vi "周期设置_采配水.vi"() -> ()   [LabVIEW 2016, in "环境动力单元.lvlib"]
uses:
  <vilib>/Utility/miscctls.llb/LVPointTypeDef.ctl
  <vilib>/Utility/config.llb/NI_LVConfig.lvlib
  <vilib>/ptbypt/NI_PtbyPt.lvlib
panel:
  in  "运行周期":T1
  # "运行模式："
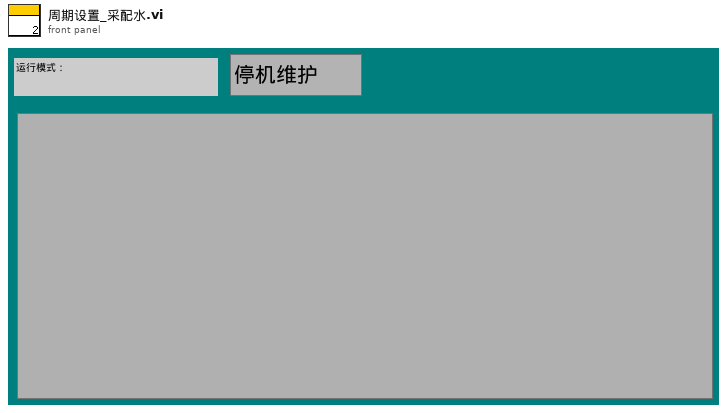
[diagram p1: front panel]
types:
  T1 = cluster{"运行模式":enum16{"停机维护", "正常运行"}, "24H周期设置":bool[]}
  T2 = typedef "LVPointTypeDef.ctl" = cluster{"Horizontal":i16, "Vertical":i16}
  T3 = typedef "NI_LVConfig.lvlib/Config Data RefNum.ctl" = refnum<k1>
  T4 = cluster{"排空时间":dbl, "润洗时间":dbl, "进样超时时间":dbl, "沉淀时间":dbl}
  T5 = typedef "LVDateTimeRec.ctl" = cluster{"秒数的小数部分":dbl, "秒":i32, "分":i32, "时":i32, "日":i32, "月":i32, "年":i32, "天数（周）":i32, "天数（年）":i32, "DST":i32}
  T6 = enum32{"Bad", "Idle", "Run top level", "Running"}
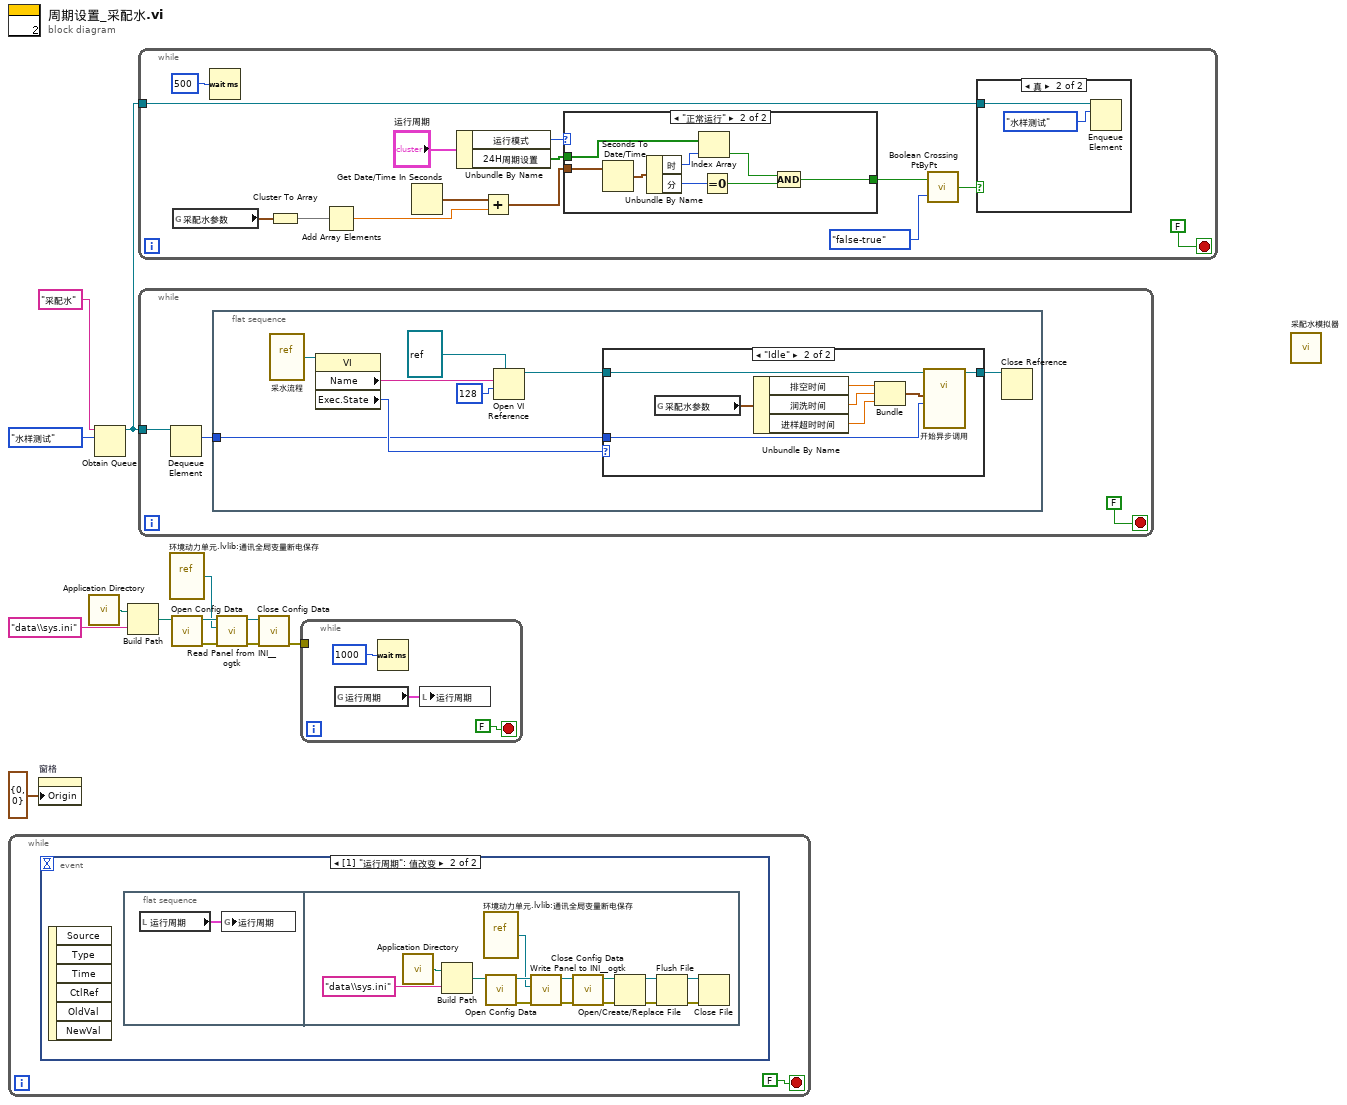
[diagram p0: block diagram]
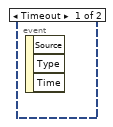
[diagram p3: hidden frame]
diagram:
  n1 = while {
    stop <- FALSE stop-if-true
    n2 = event shown="[1] \"运行周期\": 值改变" {
      selector: _ -> [_ _]
      dyn-events: _ -> [_ _]
      timeout: _ -> [_ _]
      event Timeout {
        n3 = event-data() -> ()  [unwired: 1 in, 3 out]
      }
      event "运行周期": Value Change {
        n4 = event-data() -> ()  [unwired: 1 in, 6 out]
        n5 = flat-sequence {
          frame #0 {
            n6 = local read "运行周期"() -> (w15:T1)
            n7 = global write "通讯全局变量断电保存.vi" "运行周期"(w15) -> ()
          }
          frame #1 {
            n8 = call <vilib>:"Application Directory.vi"() -> ("Application Directory"=w29:path)
            n9 = Build Path(base path=w29, name or relative path="data\\sys.ini" ("名称或相对路径")) -> (appended path=w27:path)
            n10 = vi-ref "环境动力单元.lvlib:通讯全局变量断电保存.vi"() -> (w16:refnum<vi>)
            n11 = call <vilib>:"Open Config Data.vi"("configuration file path"=w27) -> ("error out"=w24:errorcluster, "refnum"=w26:T3)  [unwired: 8 in, 1 out]
            n12 = call <userlib>:"Write Panel to INI__ogtk.vi"("error in (no error)"=w24, "VI ref"=w16, "refnum"=w26) -> ("error out"=w23:errorcluster, "refnum out"=w25:T3)  [unwired: 7 in]
            n13 = call <vilib>:"Close Config Data.vi"("error in (no error)"=w23, "refnum"=w25) -> ("error out"=w18:errorcluster, "file path"=w17:path)  [unwired: 8 in]
            n14 = Open/Create/Replace File(file path (use dialog)=w17, error in=w18) -> (refnum out=w21:refnum<file>, error out=w22:errorcluster)  [unwired: 4 in, 1 out]
            n15 = Flush File(refnum=w21, error in=w22) -> (refnum out=w20:refnum<file>, error out=w19:errorcluster)
            n16 = Close File(refnum=w20, error in=w19) -> ()  [unwired: 2 out]
          }
        }
      }
    }
  }
  n17 = property on="窗格" class="Pane"("Origin"=T2 {"Horizontal"=0, "Vertical"=0} ("原点")) -> ()  [unwired: 2 in, 2 out]
  n18 = call <vilib>:"Application Directory.vi"() -> ("Application Directory"=w7:path)
  n19 = Obtain Queue(name (unnamed)="采配水" ("名称（未命名）"), element data type=enum16{"水样测试", "加标回收"}."水样测试" ("启动类型")) -> (queue out=w1:refnum<queue>)  [unwired: 3 in, 2 out]
  n20 = Build Path(base path=w7, name or relative path="data\\sys.ini" ("名称或相对路径")) -> (appended path=w9:path)
  n21 = while {
    tunnel: w1 -> [w30]
    stop <- FALSE stop-if-true
    n22 = global read "通讯全局变量断电保存.vi" "采配水参数"() -> (w35:T4)
    n23 = Wait (ms)(milliseconds to wait=u32 500 ("等待时间（毫秒）")) -> ()  [unwired: 1 out]
    n24 = Cluster To Array(cluster=w35) -> (array=w34:dbl[])
    n25 = Add Array Elements(numeric array=w34) -> (sum=w32:dbl)
    n26 = Get Date/Time In Seconds() -> (seconds since 1Jan1904=w33:timestamp)
    n27 = Unbundle By Name("运行周期") -> ("运行模式"=w39:enum16{"停机维护", "正常运行"}, "24H周期设置"=w40:bool[])
    n28 = Add(x=w33, y=w32) -> (x+y=w31:timestamp)
    n29 = case shown="\"正常运行\"" w39 {
      tunnel: w31 -> [_ w53]
      tunnel: w40 -> [_ w50]
      tunnel: [_ w46] -> w38
      frame "停机维护", Default {
      }
      frame "正常运行" {
        n30 = Seconds To Date/Time(time stamp (now)=w53) -> (date time rec=w52:T5)  [unwired: 1 in]
        n31 = Unbundle By Name(w52) -> ("时"=w51:i32, "分"=w49:i32)
        n32 = Index Array(array=w50, index=w51) -> (element=w48:bool)
        n33 = Equal To 0?(x=w49) -> (x = 0?=w47:bool)
        n34 = Compound Arithmetic op=AND ("复合运算")(w48, w47) -> (w46:bool)
      }
    }
    n35 = call <vilib>:"Boolean Crossing PtByPt.vi"("direction"=enum16{"either", "false-true", "true-false"}."false-true", "input"=w38) -> ("crossing"=w37:bool)  [unwired: 1 in]
    n36 = case shown="真" w37 {
      tunnel: w30 -> [_ w45]
      frame False {
      }
      frame True {
        n37 = Enqueue Element(queue=w45, element=enum16{"水样测试", "加标回收"}."水样测试" ("元素")) -> ()  [unwired: 2 in, 3 out]
      }
    }
  }
  n38 = while {
    tunnel: w1 -> [w55]
    stop <- FALSE stop-if-true
    n39 = Dequeue Element(queue=w55) -> (element=w54:enum16{"水样测试", "加标回收"})  [unwired: 2 in, 3 out]
    n40 = flat-sequence {
      tunnel: w54 -> [w57]
      frame #0 {
        n41 = vi-ref "采水流程.vi"() -> (w64:refnum<vi>)
        n42 = property class="VI"(reference=w64) -> ("Name"=w60:string, "Exec.State"=w62:T6)  [unwired: 1 in, 2 out]
        n43 = Open VI Reference(type specifier VI Refnum (for type only)=refnum<vi> refnum, vi path=w60, options=128 ("选项")) -> (vi reference=w59:refnum<vi>)  [unwired: 3 in, 1 out]
        n44 = case shown="\"Idle\"" w62 {
          tunnel: [w65 w73] -> w63
          tunnel: w59 -> [w65 w72]
          tunnel: w57 -> [_ w66]
          frame "Bad", Default {
          }
          frame "Idle" {
            n45 = global read "通讯全局变量断电保存.vi" "采配水参数"() -> (w71:T4)
            n46 = Unbundle By Name(w71) -> ("排空时间"=w70:dbl, "润洗时间"=w69:dbl, "进样超时时间"=w68:dbl)
            n47 = Bundle("排空时间"=w70, "润洗时间"=w69, "进样超时时间"=w68) -> (w67:cluster{"排空时间":dbl, "润洗时间":dbl, "进样超时时间":dbl})  [unwired: 1 in]
            n48 = call-by-ref "开始异步调用"(reference=w72, "启动类型"=w66, "参数设置"=w67) -> (reference out=w73:refnum<vi>)  [unwired: 11 in, 1 out]
          }
        }
        n49 = Close Reference(reference=w63) -> ()  [unwired: 1 in, 1 out]
      }
    }
  }
  n50 = vi-ref "环境动力单元.lvlib:通讯全局变量断电保存.vi"() -> (w4:refnum<vi>)
  n51 = call <vilib>:"Open Config Data.vi"("configuration file path"=w9) -> ("error out"=w12:errorcluster, "refnum"=w10:T3)  [unwired: 8 in, 1 out]
  n52 = call <userlib>:"Read Panel from INI__ogtk.vi"("error in (no error)"=w12, "VI ref"=w4, "refnum"=w10) -> ("error out"=w13:errorcluster, "refnum out"=w11:T3)  [unwired: 7 in]
  n53 = call <vilib>:"Close Config Data.vi"("error in (no error)"=w13, "refnum"=w11) -> ("error out"=w6:errorcluster)  [unwired: 8 in, 1 out]
  n54 = while {
    tunnel: w6 -> [_]
    stop <- FALSE stop-if-true
    n55 = global read "通讯全局变量断电保存.vi" "运行周期"() -> (w74:T1)
    n56 = Wait (ms)(milliseconds to wait=u32 1000 ("等待时间（毫秒）")) -> ()  [unwired: 1 out]
    n57 = local write "运行周期"(w74) -> ()
  }
  n58 = call "采配水模拟器.vi"() -> ()  [unwired: 12 in]
